vi "Save Suite to Index.vi"(8 "error in (no error)":errorcluster, 10 "Suite":refnum<class "LUnit Test Suite.lvclass">, 11 "Test Finder In":refnum<class "Test Finder.lvclass">) -> (0 "error out":errorcluster)   [LabVIEW 2020, in "Test Finder.lvclass"]
uses:
  Test Finder.lvclass
  LUnit Test Suite.lvclass
  Test Finder.lvclass/Test Finder.ctl
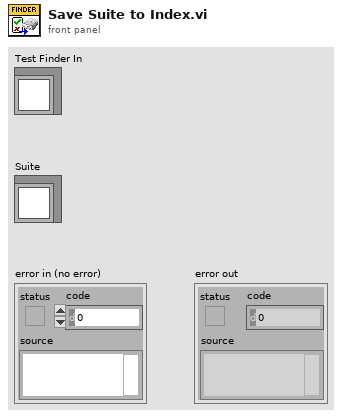
[diagram p1: front panel]
types:
  T1 = enum16{"open", "replace", "create", "open or create", "replace or create", "replace or create with confirmation"}
  T2 = typedef "Test Finder.lvclass/Index.ctl" = cluster{"Checksums":map{path, string}, "Suite":refnum<class "LUnit Test Suite.lvclass">}
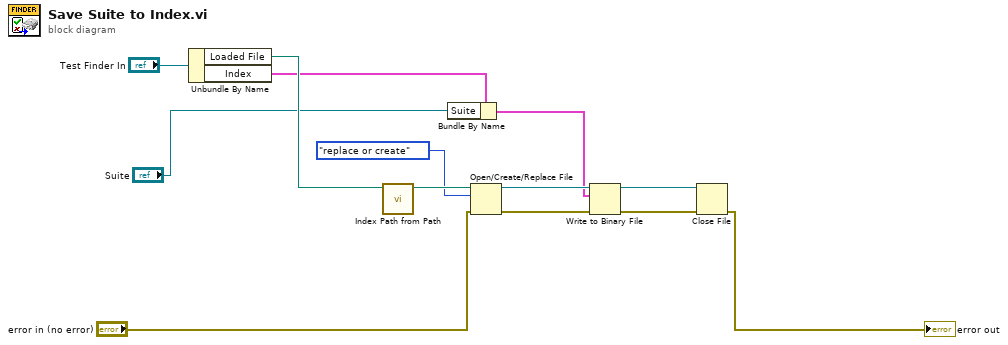
[diagram p0: block diagram]
diagram:
  n1 = Unbundle By Name("Test Finder In") -> ("Loaded File"=w8:path, "Index"=w7:T2)
  n2 = call "Index Path from Path.vi"("Project Path"=w8) -> ("appended path"=w13:path)  [unwired: 10 in]
  n3 = Bundle By Name(cluster=w7, "Suite"="Suite") -> (w5:T2)
  n4 = Open/Create/Replace File(file path (use dialog)=w13, error in="error in (no error)", operation (0:open)=T1."replace or create") -> (refnum out=w12:refnum<file>, error out=w4:errorcluster)  [unwired: 3 in, 1 out]
  n5 = Write to Binary File(file (use dialog)=w12, data=w5, error in=w4) -> (refnum out=w11:refnum<file>, error out=w3:errorcluster)  [unwired: 3 in, 1 out]
  n6 = Close File(refnum=w11, error in=w3) -> (error out=→"error out":errorcluster)  [unwired: 1 out]
